vi "imprimer etiquette.vi"(0 "chaine à écrire":string="^XA\n^KL3\n^SC9600,8,N,1,,N\n^PRA\n^LL976\n^ML592\n^LH50,25\r\r^ADB,1,1^FT25,704^FDKunde:Fluid Automat. Systems GmbH^FS\r^ADB,1,1^FT50,704^FDBestellnummer:120077 / 109654     ^FS\r^ADB,1,1^FT75,704^FDKarton:1/4^FS\r^ADB,1,1^FT100,704^FDAnzahl:25/100^FS\r^ADB,1,1^FT125,704^FDIhre Art.-Nr.: MK01852 ^FS\r^ADB,1,1^FT180,704^FDVentil-Nr.:^FS\r^ADB,1,1^FT205,678^FD(P/N)^FS\r\r^FT408,40\n^BY1,2.0\n^BCI,56,N,N,N\n^FD MK01852  09 ARZAARZA 25^FS\r^AQI,1,1^FT408,10^FD MK01852  09 ARZAARZA 25^FS\r\r^A0B,18,18^FT180,568^FD ARZA6051,  ARZA6052,  ARZA6053,  ARZA6054^FS\r^A0B,18,18^FT198,568^FD ARZA6055,  ARZA6056,  ARZA6057,  ARZA6058^FS\r^A0B,18,18^FT216,568^FD ARZA6059,  ARZA6060,  ARZA6061,  ARZA6062^FS\r^A0B,18,18^FT234,568^FD ARZA6063,  ARZA6064,  ARZA6065,  ARZA6066^FS\r^A0B,18,18^FT252,568^FD ARZA6067,  ARZA6068,  ARZA6069,  ARZA6070^FS\r^A0B,18,18^FT270,568^FD ARZA6071,  ARZA6072,  ARZA6073,  ARZA6074 ^FS\r^A0B,18,18^FT288,568^FD ARZA6075 ^FS\r^A0B,18,18^FT306,568^FD ^FS\r^A0B,18,18^FT324,568^FD ^FS\r^A0B,18,18^FT242,568^FD ^FS\r\r^FT370,708\n^GB0,565,3^FS\n\n^FT501,708\n^BXB,4,0\n^FD01-223E-01-B6 F011107 18V DC 4.5W     R01159/08-01.01.01^FS\r^ADB,1,1^FT413,568^FDFAS Artikelnummer:^FS\r^AQB,1,1^FT443,568^FD01-223E-01-B6 F011107 18V DC 4.5W^FS\r^ADB,1,1^FT470,568^FDFAS Bestellnummer:^FS\r^AQB,1,1^FT500,568^FDR01159/08-01.01.01^FS\r\r^PQ1\n^XZ\r", 1 "nbr de valve":i16=10, 2 "nbr de carton":i16=1, 4 "Type de liaison":enum16{"RS232", "USB", "TCP-IP", "Aucune"}(ring)=enum."TCP-IP", 6 "Bloc Scanné":string, 7 "n°article FAS":string, 9 "sélecteur":bool, 10 "Cde_Interne":bool, 11 "error in":errorcluster caption="entrée d'erreur (pas d'erreur)", 13 "Carton Numéro":i16, 14 "fin de série ?":bool) -> (15 "error out":errorcluster caption="sortie d'erreur")   [LabVIEW 2020]
uses:
  Labview emballage/enum_ON_OFF_Lecteur.ctl
  Modules/FS/60_FS_Controles/60_FS_SetGet.ctl
  <vilib>/Instr/_visa.llb/VISA Configure Serial Port (Instr).vi
panel:
  in  "Msg Etiquette imprimée":string="L'étiquette est-elle correctement\nimprimée ?"
  out "Etiquette scanné":string
  out "Série finie":string="Il y a 1 carton(s)"
  out "Changer de carton":string="Il y a 1 carton(s)"
  out "Nbre de valve":string="pour 10 valves/blocs"
  out "Nbre de carton":string="Il y a 1 carton(s)"
  out "Carton No :":string
  out "Glissière 2":u8(slide)=100 caption="Identification terminé." scale=0.0..100.0
  in  "ré-imprimer":bool
  in  "Bouton confirmer":bool
  in  "Nom de ressource VISA USB":refnum<visa-resource-name>
  in  "Param RS232":T1={"VISA resource name"="COM4", "baud rate"=9600, "data bits"=8, "parity"=0, "stop bits"=10, "flow control"=0, "delay before read (ms)"=500} {"data bits" min=5 max=8 step=1; "parity" items=["Aucune", "Impaire", "Paire", "Marque", "Espace"]; "stop bits" items=["1.0"=10, "1.5"=15, "2.0"=20]; "flow control" items=["Aucune"=0, "XON/XOFF"=1, "RTS/CTS"=2, "DTR/DSR"=4]}
  # "LOGO FASmedic en noir et blanc"
  # "Uniquement par un responsable"
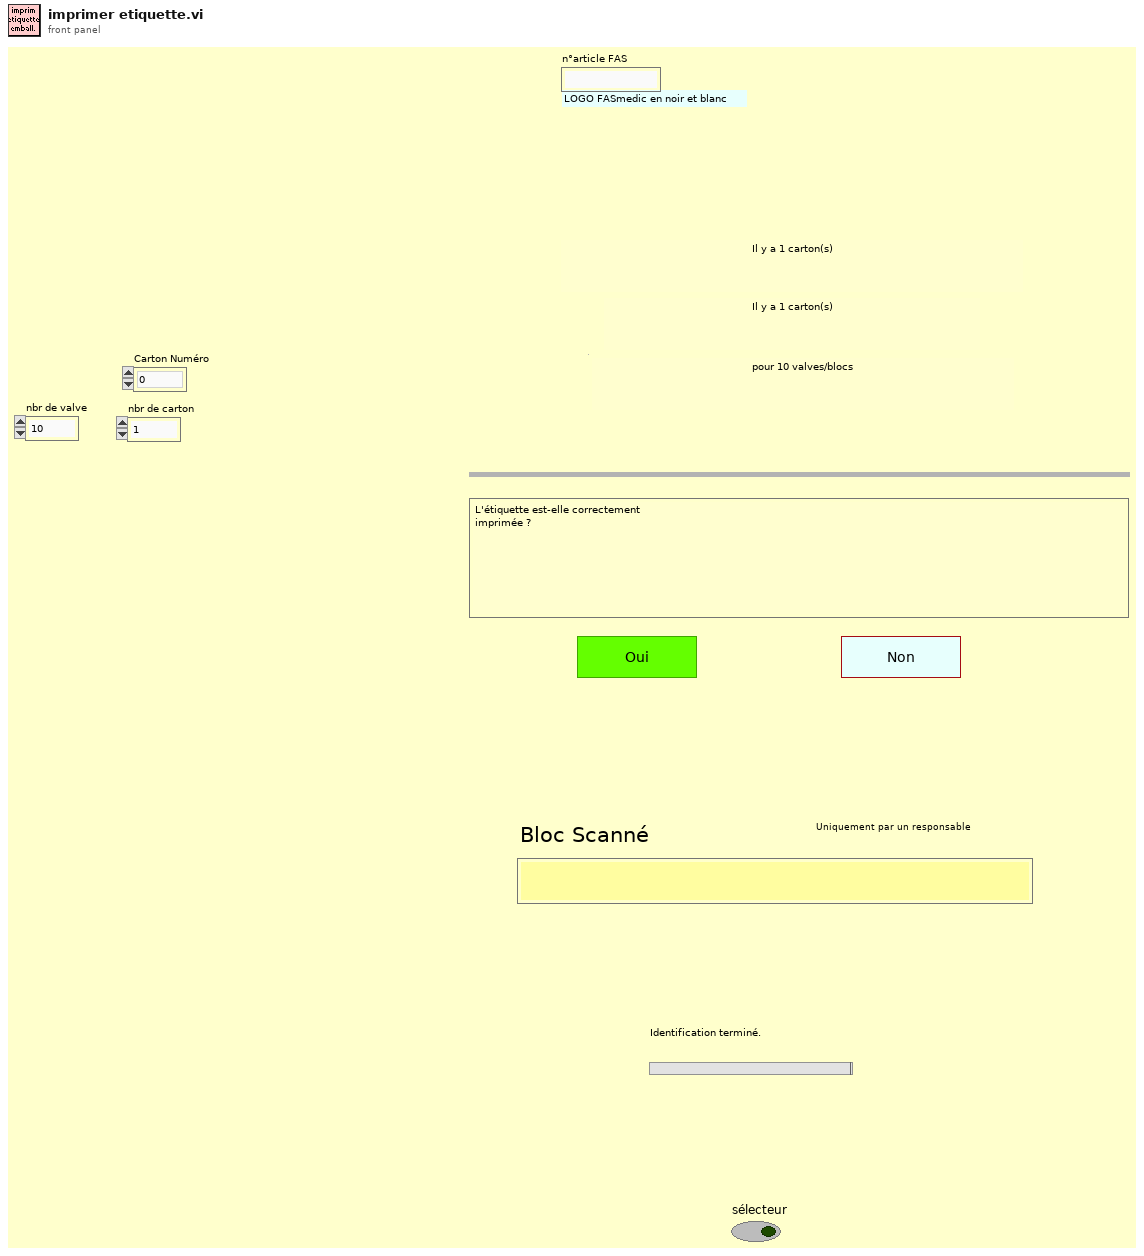
[diagram p1: front panel]
types:
  T1 = cluster{"VISA resource name":refnum<visa-resource-name>, "baud rate":u32, "data bits":u16, "parity":u16, "stop bits":u16, "flow control":u16, "delay before read (ms)":u32}
  T2 = typedef "enum_ON_OFF_Lecteur.ctl" = enum16{"ON_COURT", "OFF", "ON", "OFF (open/Close)", "ON (open/close)"}
  T3 = typedef "60_FS_SetGet.ctl" = enum16{"set", "get"}
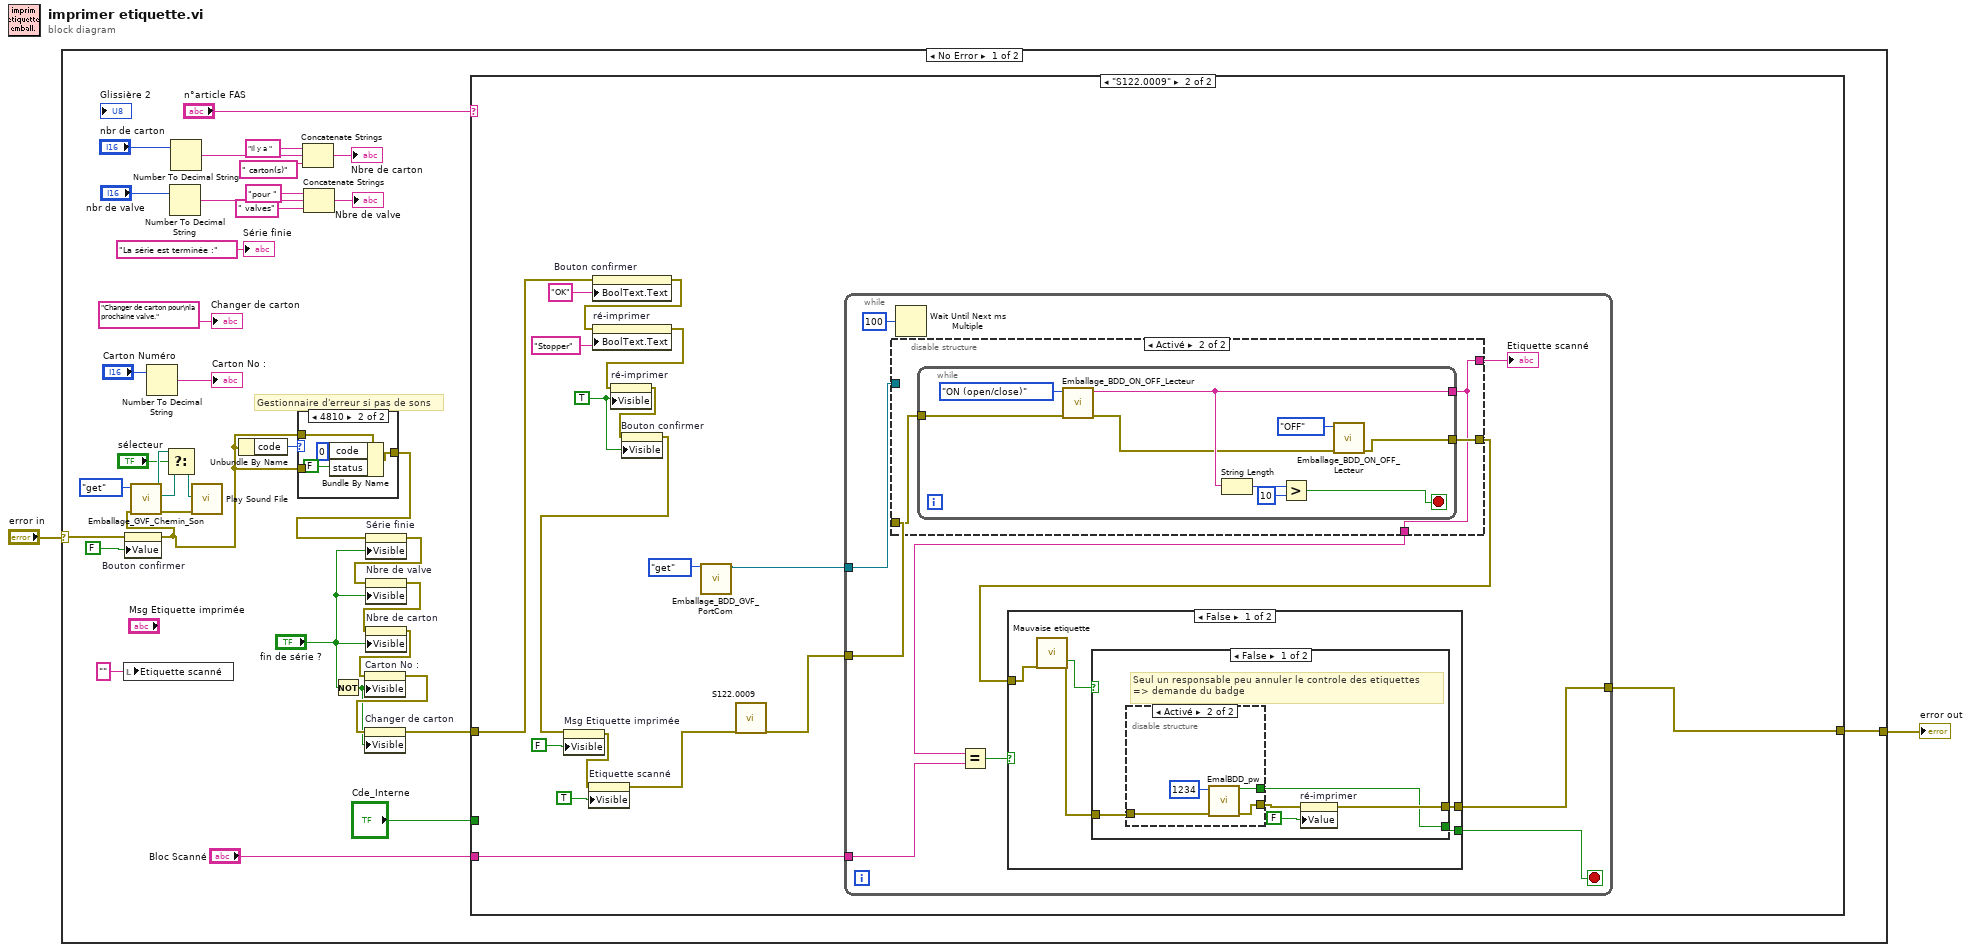
[diagram p0: block diagram]
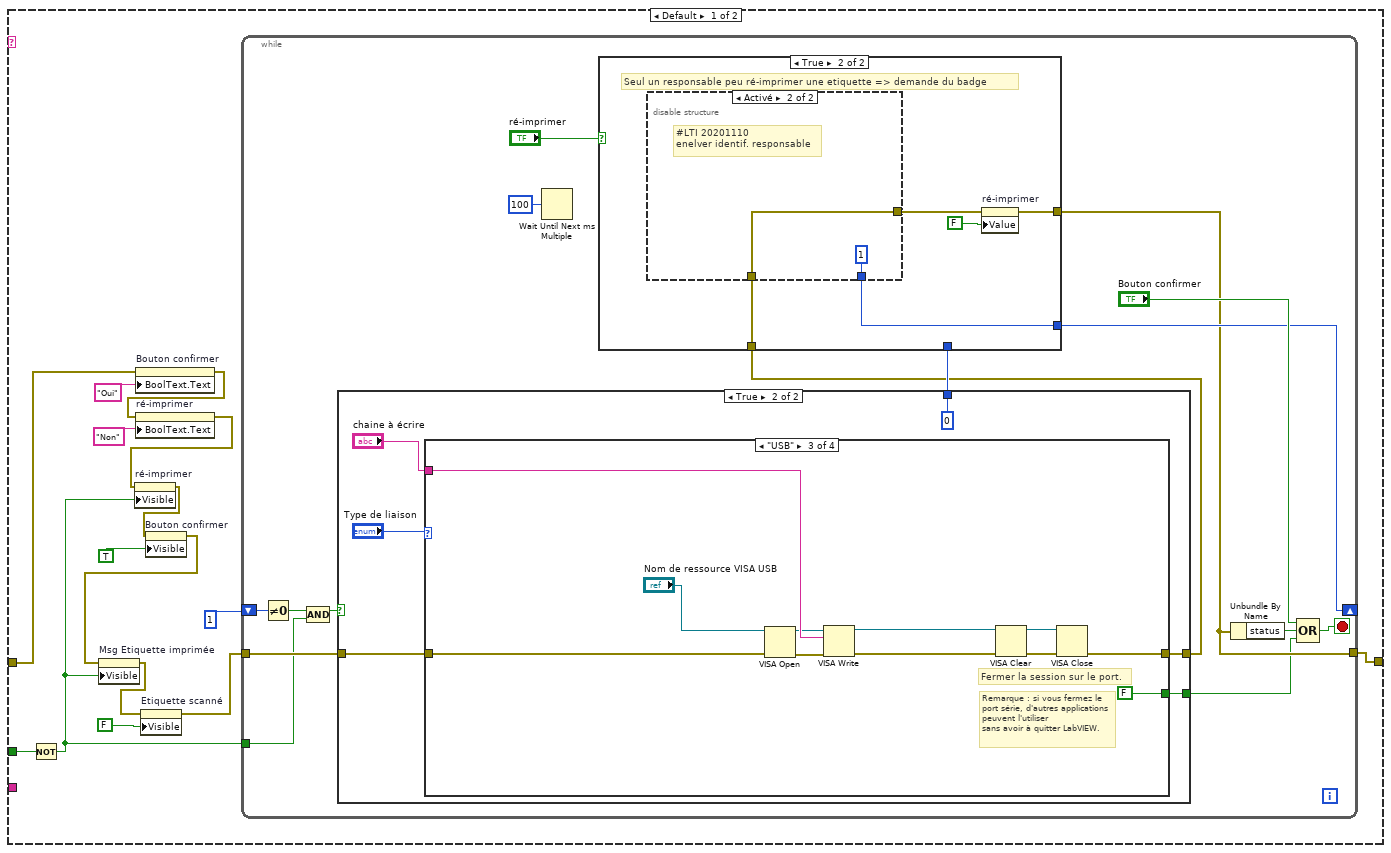
[diagram p2: hidden frame]
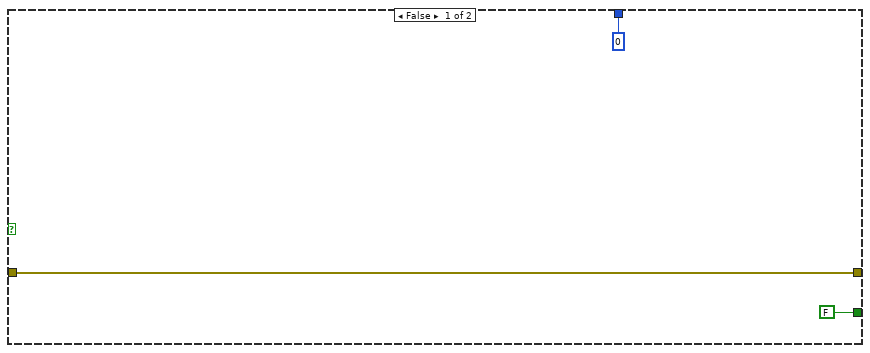
[diagram p3: hidden frame]
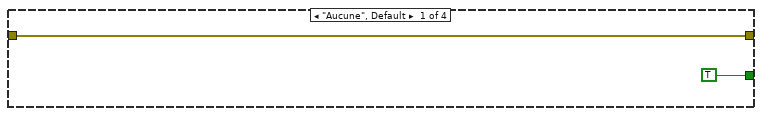
[diagram p4: hidden frame]
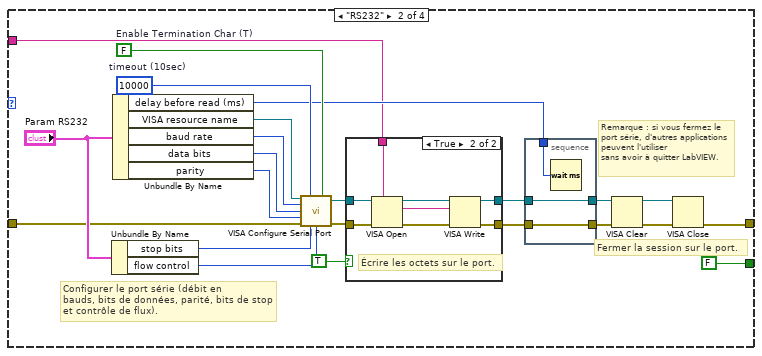
[diagram p5: hidden frame]
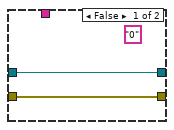
[diagram p6: hidden frame]
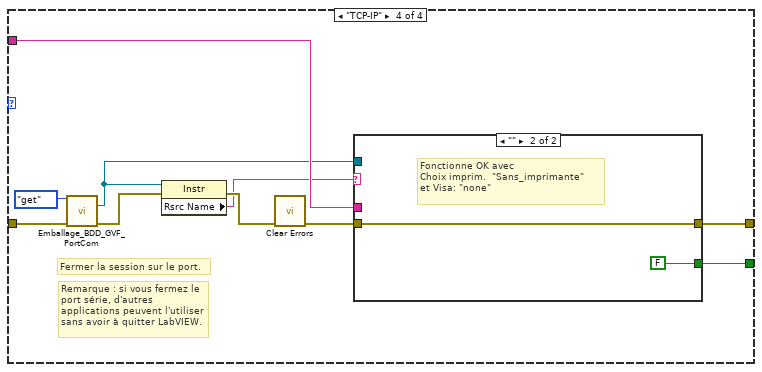
[diagram p7: hidden frame]
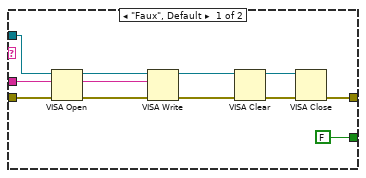
[diagram p8: hidden frame]
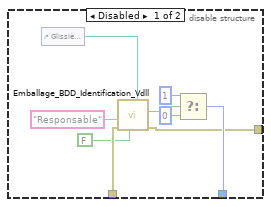
[diagram p10: hidden frame]
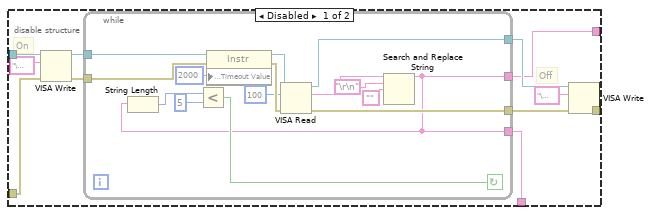
[diagram p11: hidden frame]
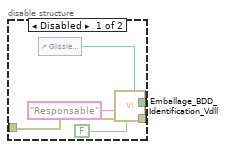
[diagram p12: hidden frame]
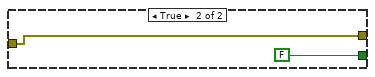
[diagram p13: hidden frame]
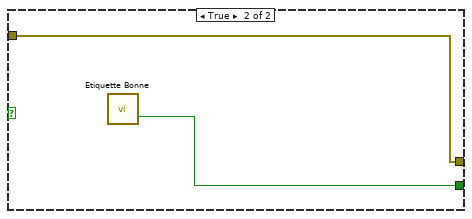
[diagram p14: hidden frame]
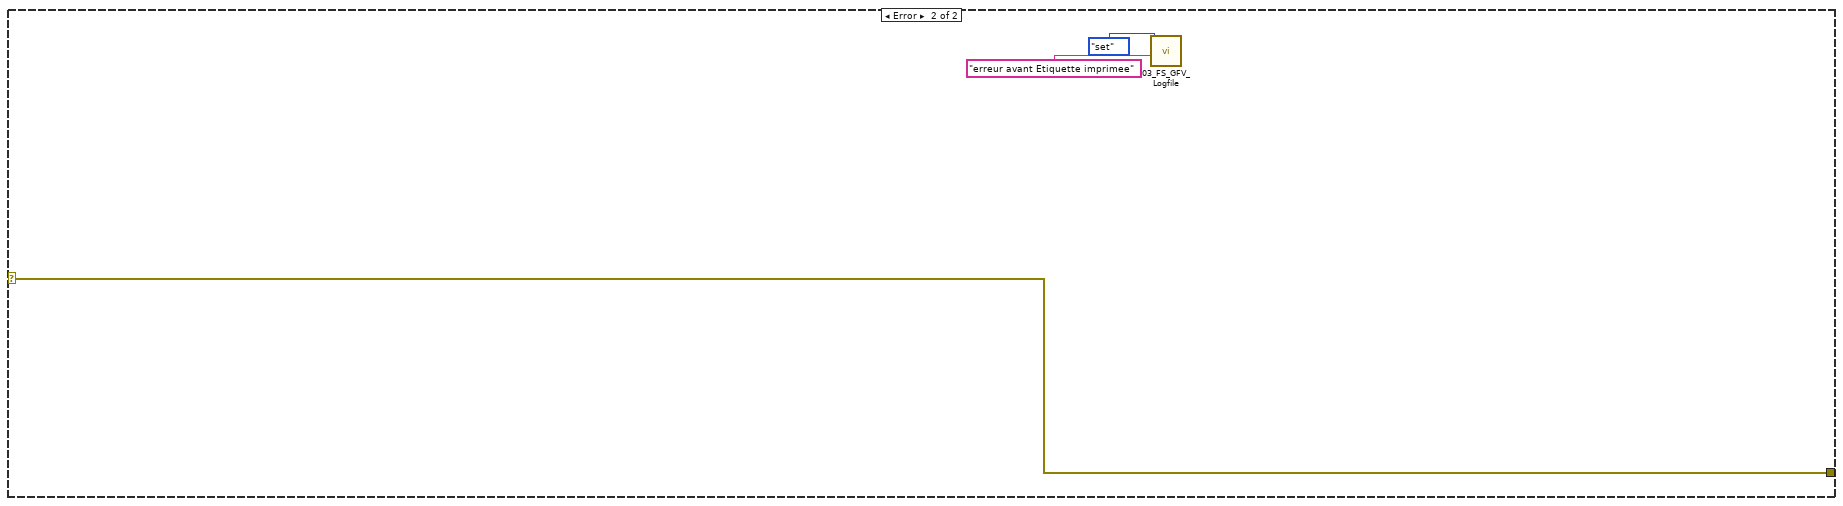
[diagram p16: hidden frame]
diagram:
  n1 = case shown="No Error" "error in" {
    selector: "error in" -> [w38 w264]
    tunnel: [w39 w264] -> w1
    frame No Error {
      # "Gestionnaire d'erreur si pas de sons"
      n2 = local write "Etiquette scanné"("" ("Numéro scanné")) -> ()
      n3 = property on="Bouton confirmer" class="Bool (strict)"(error in=w38, "Value"=FALSE ("Bouton confimer")) -> (error out=w7:errorcluster)  [unwired: 1 in, 1 out]
      n4 = call "Emballage_GVF_Chemin_Son.vi"("entrée d'erreur (pas d'erreur)"=w7, "Énum"=enum16{"get", "set"}."get") -> ("sortie d'erreur"=w8:errorcluster, "Chemin Utopia - Question.WAV"=w4:path, "Chemin The Microsoft Sound.wav"=w5:path)  [unwired: 5 in, 2 out]
      n5 = Number To Decimal String(number="Carton Numéro") -> (decimal integer string=→"Carton No :":string)  [unwired: 1 in]
      n6 = Select(t=w5, s="sélecteur", f=w4) -> (s? t:f=w6:path)
      n7 = Number To Decimal String(number="nbr de valve") -> (decimal integer string=w34:string)  [unwired: 1 in]
      n8 = Number To Decimal String(number="nbr de carton") -> (decimal integer string=w30:string)  [unwired: 1 in]
      n9 = call <vilib>:"Play Sound File.vi"("error in (no error)"=w8, "path"=w6) -> ()  [unwired: 8 in, 2 out]
      n10 = Unbundle By Name(w7) -> ("code"=w15:i32)
      n11 = case shown="4810" w15 {
        tunnel: [w257 w260] -> w14
        tunnel: w7 -> [w257 _]
        tunnel: w7 -> [_ w259]
        frame 0, Default {
        }
        frame 4810 {
          n12 = Bundle By Name(cluster=w259, "code"=0, "status"=FALSE) -> (w260:errorcluster)
        }
      }
      n13 = Concatenate Strings("Il y a ", w30, " carton(s)") -> (→"Nbre de carton":string)
      n14 = Concatenate Strings("pour ", w34, " valves") -> (→"Nbre de valve":string)
      n15 = Not(x="fin de série ?") -> (.not. x?=w19:bool)
      n16 = property on="Série finie" class="Str"(error in=w14, "Visible"="fin de série ?") -> (error out=w16:errorcluster)  [unwired: 1 in, 1 out]
      n17 = property on="Nbre de valve" class="Str"(error in=w16, "Visible"="fin de série ?") -> (error out=w26:errorcluster)  [unwired: 1 in, 1 out]
      n18 = property on="Nbre de carton" class="Str"(error in=w26, "Visible"="fin de série ?") -> (error out=w25:errorcluster)  [unwired: 1 in, 1 out]
      n19 = property on="Carton No :" class="Str"(error in=w25, "Visible"=w19) -> (error out=w23:errorcluster)  [unwired: 1 in, 1 out]
      n20 = property on="Changer de carton" class="Str"(error in=w23, "Visible"=w19) -> (error out=w22:errorcluster)  [unwired: 1 in, 1 out]
      n21 = case shown="\"S122.0009\"" "n°article FAS" {
        tunnel: [w54 w179] -> w39
        tunnel: w22 -> [w43 w172]
        tunnel: "Bloc Scanné" -> [_ w170]
        tunnel: "Cde_Interne" -> [w41 _]
        frame Default {
          n22 = Not(x=w41) -> (.not. x?=w40:bool)
          n23 = property on="Bouton confirmer" class="Bool (strict)"(error in=w43, "BoolText.Text"="Oui" ("Texte booléen.Texte")) -> (error out=w44:errorcluster)  [unwired: 1 in, 1 out]
          n24 = property on="ré-imprimer" class="Bool (strict)"(error in=w44, "BoolText.Text"="Non" ("Texte booléen.Texte")) -> (error out=w42:errorcluster)  [unwired: 1 in, 1 out]
          n25 = property on="ré-imprimer" class="Bool (strict)"(error in=w42, "Visible"=w40) -> (error out=w49:errorcluster)  [unwired: 1 in, 1 out]
          n26 = property on="Bouton confirmer" class="Bool (strict)"(error in=w49, "Visible"=TRUE) -> (error out=w47:errorcluster)  [unwired: 1 in, 1 out]
          n27 = property on="Msg Etiquette imprimée" class="Str"(error in=w47, "Visible"=w40) -> (error out=w51:errorcluster)  [unwired: 1 in, 1 out]
          n28 = property on="Etiquette scanné" class="Str"(error in=w51, "Visible"=FALSE) -> (error out=w50:errorcluster)  [unwired: 1 in, 1 out]
          n29 = while {
            tunnel: w50 -> [w69]
            tunnel: [w58] -> w54
            shift-right: [w60] -> _
            shift-left: u32 1 ("n millisecondes") -> [w62]
            tunnel: w40 -> [w55]
            stop <- w64 stop-if-true
            n30 = Not Equal To 0?(x=w62) -> (x != 0?=w63:bool)
            n31 = Compound Arithmetic op=AND(w63, w55) -> (w56:bool)
            n32 = case shown="True" w56 {
              tunnel: w69 -> [w72 w78]
              tunnel: [w72 w76] -> w59
              tunnel: [u32 0 ("n millisecondes") u32 0 ("n millisecondes")] -> w61
              tunnel: [FALSE w74] -> w57
              frame False {
              }
              frame True {
                n33 = case shown="\"USB\"" "Type de liaison" {
                  tunnel: w78 -> [w80 w88 w120 w131]
                  tunnel: [w80 w82 w121 w135] -> w76
                  tunnel: "chaine à écrire" -> [_ w87 w126 w136]
                  tunnel: [TRUE FALSE FALSE w132] -> w74
                  frame "Aucune", Default {
                  }
                  frame "RS232" {
                    w102 = FALSE  # Enable Termination Char (T)
                    w103 = u32 10000  # timeout (10sec)
                    # "Remarque : si vous fermez le port série, d'autres applications peuvent l'utiliser\nsans avoir à quitter LabVIEW."
                    # "Fermer la session sur le port."
                    # "Configurer le port série (débit en\nbauds, bits de données, parité, bits de stop\net contrôle de flux)."
                    n34 = Unbundle By Name("Param RS232") -> ("stop bits"=w96:u16, "flow control"=w95:u16)
                    n35 = Unbundle By Name("Param RS232") -> ("delay before read (ms)"=w91:u32, "VISA resource name"=w101:refnum<visa-resource-name>, "baud rate"=w100:u32, "data bits"=w99:u16, "parity"=w98:u16)
                    n36 = call-poly "VISA Configure Serial Port"("VISA resource name"=w101, "timeout (10sec)"=w103, "Enable Termination\nChar (T)"=w102, "baud rate (9600)"=w100, "data bits (8)"=w99, "parity (0:none)"=w98, "error in (no error)"=w88, "stop bits (10: 1 bit)"=w96, "flow control (0:none)"=w95) -> ("VISA resource name out"=w90:refnum<visa-resource-name>, "error out"=w89:errorcluster)  [unwired: 5 in]
                    n37 = case shown="True" TRUE {
                      tunnel: [w108 w115] -> w94
                      tunnel: w90 -> [w107 w114]
                      tunnel: w89 -> [w108 w110]
                      tunnel: [w107 w113] -> w93
                      tunnel: w87 -> [_ w112]
                      frame False {
                        (unwired) "0" ("string to write")
                      }
                      frame True {
                        # "Écrire les octets sur le port."
                        n38 = VISA Open(error in (no error)=w110, VISA resource name=w114) -> (VISA resource name=w111:refnum<visa-resource-name>, error out=w109:errorcluster)  [unwired: 3 in]
                        n39 = VISA Write(VISA resource name=w111, write buffer=w112, error in (no error)=w109) -> (VISA resource name out=w113:refnum<visa-resource-name>, error out=w115:errorcluster)  [unwired: 1 out]
                      }
                    }
                    n40 = stacked-sequence {
                      tunnel: w94 -> [w106]
                      tunnel: [w106] -> w84
                      tunnel: w93 -> [w105]
                      tunnel: [w105] -> w83
                      tunnel: w91 -> [w104]
                      frame #0 {
                        n41 = Wait (ms)(milliseconds to wait=w104) -> ()  [unwired: 1 out]
                      }
                    }
                    n42 = VISA Clear(VISA resource name=w83, error in (no error)=w84) -> (VISA resource name out=w85:refnum<visa-resource-name>, error out=w86:errorcluster)
                    n43 = VISA Close(VISA resource name=w85, error in (no error)=w86) -> (error out=w82:errorcluster)
                  }
                  frame "USB" {
                    # "Remarque : si vous fermez le port série, d'autres applications peuvent l'utiliser\nsans avoir à quitter LabVIEW."
                    # "Fermer la session sur le port."
                    n44 = VISA Open(error in (no error)=w120, VISA resource name="Nom de ressource VISA USB") -> (VISA resource name=w118:refnum<visa-resource-name>, error out=w117:errorcluster)  [unwired: 3 in]
                    n45 = VISA Write(VISA resource name=w118, write buffer=w126, error in (no error)=w117) -> (VISA resource name out=w122:refnum<visa-resource-name>, error out=w123:errorcluster)  [unwired: 1 out]
                    n46 = VISA Clear(VISA resource name=w122, error in (no error)=w123) -> (VISA resource name out=w124:refnum<visa-resource-name>, error out=w125:errorcluster)
                    n47 = VISA Close(VISA resource name=w124, error in (no error)=w125) -> (error out=w121:errorcluster)
                  }
                  frame "TCP-IP" {
                    # "Remarque : si vous fermez le port série, d'autres applications peuvent l'utiliser\nsans avoir à quitter LabVIEW."
                    # "Fermer la session sur le port."
                    n48 = call "Emballage_BDD_GVF_PortCom.vi"("Énum"=enum16{"get", "set"}."get", "Error in"=w131) -> ("PortCom imprimante OUT"=w128:refnum<visa-resource-name>, "Error out"=w130:errorcluster)  [unwired: 7 in, 5 out]
                    n49 = property class="Instr"(reference=w128, error in=w130) -> (error out=w134:errorcluster, "Rsrc Name"=w127:string)  [unwired: 1 out]
                    n50 = call <vilib>:"Clear Errors.vi"("error in (no error)"=w134) -> ("error out"=w133:errorcluster)  [unwired: 5 in, 1 out]
                    n51 = case shown="\"\"" w127 {
                      tunnel: w136 -> [w147 _]
                      tunnel: [w142 w149] -> w135
                      tunnel: w133 -> [w140 w149]
                      tunnel: w128 -> [w138 _]
                      tunnel: [FALSE FALSE] -> w132
                      frame "Faux", Default {
                        n52 = VISA Open(error in (no error)=w140, VISA resource name=w138) -> (VISA resource name=w141:refnum<visa-resource-name>, error out=w139:errorcluster)  [unwired: 3 in]
                        n53 = VISA Write(VISA resource name=w141, write buffer=w147, error in (no error)=w139) -> (VISA resource name out=w143:refnum<visa-resource-name>, error out=w144:errorcluster)  [unwired: 1 out]
                        n54 = VISA Clear(VISA resource name=w143, error in (no error)=w144) -> (VISA resource name out=w145:refnum<visa-resource-name>, error out=w146:errorcluster)
                        n55 = VISA Close(VISA resource name=w145, error in (no error)=w146) -> (error out=w142:errorcluster)
                      }
                      frame "" {
                        # "Fonctionne OK avec \nChoix imprim.  \"Sans_imprimante\"\net Visa: \"none\""
                      }
                    }
                  }
                }
              }
            }
            n56 = Wait Until Next ms Multiple(millisecond multiple=u32 100 ("n millisecondes")) -> ()  [unwired: 1 out]
            n57 = case shown="True" "ré-imprimer" {
              tunnel: w61 -> [w151 _]
              tunnel: [w151 w156] -> w60
              tunnel: w59 -> [w150 w155]
              tunnel: [w150 w154] -> w58
              frame False {
              }
              frame True {
                # "Seul un responsable peu ré-imprimer une etiquette => demande du badge"
                n58 = disable-structure shown="Activé" {
                  disable-tunnel: [w162 u32 1 ("cas faux")] -> w156
                  disable-tunnel: w155 -> [w160 w166]
                  disable-tunnel: [w157 w166] -> w153
                  frame Disabled {
                    n59 = control-ref of="Glissière 2"() -> (w158:refnum<vi>)
                    n60 = call "Emballage_BDD_Identification_Vdll.vi"("Glissière"=w158, "lecture seul possible ?"=FALSE, "error in"=w160, "Posage choisi"="Responsable" ("Posage choissi")) -> ("error Out"=w157:errorcluster, "OK"=w164:bool)  [unwired: 3 in, 3 out]
                    n61 = Select(t=u32 1 ("n millisecondes"), s=w164, f=u32 0 ("cas faux")) -> (s? t:f=w162:u32)
                  }
                  frame Enabled {
                    # "#LTI 20201110\nenelver identif. responsable"
                  }
                }
                n62 = property on="ré-imprimer" class="Bool (strict)"(error in=w153, "Value"=FALSE ("ré-imprimer")) -> (error out=w154:errorcluster)  [unwired: 1 in, 1 out]
              }
            }
            n63 = Unbundle By Name(w58) -> ("status"=w66:bool)
            n64 = Compound Arithmetic op=OR("Bouton confirmer", w66, w57) -> (w64:bool)
          }
        }
        frame "S122.0009" {
          w178 = TRUE ("Visible")
          n65 = property on="Bouton confirmer" class="Bool (strict)"(error in=w172, "BoolText.Text"="OK" ("Texte booléen.Texte")) -> (error out=w173:errorcluster)  [unwired: 1 in, 1 out]
          n66 = property on="ré-imprimer" class="Bool (strict)"(error in=w173, "BoolText.Text"="Stopper" ("Texte booléen.Texte")) -> (error out=w171:errorcluster)  [unwired: 1 in, 1 out]
          n67 = property on="ré-imprimer" class="Bool (strict)"(error in=w171, "Visible"=w178) -> (error out=w177:errorcluster)  [unwired: 1 in, 1 out]
          n68 = property on="Bouton confirmer" class="Bool (strict)"(error in=w177, "Visible"=w178) -> (error out=w176:errorcluster)  [unwired: 1 in, 1 out]
          n69 = property on="Msg Etiquette imprimée" class="Str"(error in=w176, "Visible"=FALSE) -> (error out=w182:errorcluster)  [unwired: 1 in, 1 out]
          n70 = property on="Etiquette scanné" class="Str"(error in=w182, "Visible"=TRUE) -> (error out=w181:errorcluster)  [unwired: 1 in, 1 out]
          n71 = call "Emballage_BDD_GVF_PortCom.vi"("Énum"=enum16{"get", "set"}."get") -> ("PortCom Scanner"=w168:refnum<visa-resource-name>)  [unwired: 8 in, 6 out]
          n72 = call "S122.0009"("error in (no error)"=w181) -> ("error out"=w180:errorcluster)  [unwired: 17 in, 1 out]
          n73 = while {
            tunnel: w168 -> [w194]
            tunnel: w180 -> [w193]
            tunnel: [w187] -> w179
            tunnel: w170 -> [w192]
            stop <- w188 stop-if-true
            n74 = disable-structure shown="Activé" {
              disable-tunnel: w194 -> [w205 _]
              disable-tunnel: w193 -> [w204 w223]
              disable-tunnel: [w197 w221] -> w191
              disable-tunnel: [w196 w222] -> w186
              disable-tunnel: [w195 w221] -> w185
              frame Disabled {
                # "Off"
                # "On"
                n75 = VISA Write(VISA resource name=w205, write buffer="\u0002", error in (no error)=w204) -> (VISA resource name out=w202:refnum<visa-resource-name>, error out=w203:errorcluster)  [unwired: 1 out]
                n76 = while {
                  tunnel: [w220] -> w198
                  tunnel: w203 -> [w212]
                  tunnel: w202 -> [w211]
                  tunnel: [w207] -> w199
                  tunnel: [w206] -> w197
                  tunnel: [w206] -> w195
                  stop <- w208 continue-if-true
                  n77 = property class="Instr"(reference=w211, error in=w212, "General Settings:Timeout Value"=u32 2000 ("Tmo Value")) -> (reference out=w218:refnum<visa-resource-name>, error out=w219:errorcluster)
                  n78 = VISA Read(VISA resource name=w218, byte count=u32 100 ("byte count (0)"), error in (no error)=w219) -> (VISA resource name out=w207:refnum<visa-resource-name>, read buffer=w215:string, error out=w220:errorcluster)  [unwired: 1 out]
                  n79 = Search and Replace String(input string=w215, search string="\r\n", replace string="") -> (result string=w206:string)  [unwired: 5 in, 3 out]
                  n80 = String Length(string=w206) -> (length=w210:i32)
                  n81 = Less?(x=w210, y=5) -> (x < y?=w208:bool)
                }
                n82 = VISA Write(VISA resource name=w199, write buffer="\u0003", error in (no error)=w198) -> (error out=w196:errorcluster)  [unwired: 2 out]
              }
              frame Enabled {
                n83 = while {
                  tunnel: w223 -> [w231]
                  tunnel: [w228] -> w221
                  tunnel: [w226] -> w222
                  stop <- w227 stop-if-true
                  n84 = call "Emballage_BDD_ON_OFF_Lecteur.vi"("Error in"=w231, "ON/OFF lecteur"=enum_ON_OFF_Lecteur."ON (open/close)") -> ("Error out"=w225:errorcluster, "Etiquette scanné"=w228:string)  [unwired: 7 in, 1 out]
                  n85 = String Length(string=w228) -> (length=w229:i32)
                  n86 = Greater?(x=w229, y=10) -> (0:w227:bool)
                  n87 = call "Emballage_BDD_ON_OFF_Lecteur.vi"("Error in"=w225, "ON/OFF lecteur"=enum_ON_OFF_Lecteur."OFF") -> ("Error out"=w226:errorcluster)  [unwired: 7 in, 2 out]
                }
              }
            }
            "Etiquette scanné" <- w185
            n88 = Wait Until Next ms Multiple(millisecond multiple=u32 100 ("n millisecondes")) -> ()  [unwired: 1 out]
            n89 = Equal?(x=w191, y=w192) -> (x = y?=w189:bool)
            n90 = case shown="False" w189 {
              tunnel: [w233 w256] -> w188
              tunnel: [w235 w255] -> w187
              tunnel: w186 -> [w234 w255]
              frame False {
                n91 = call "Mauvaise etiquette"("error in (no error)"=w234) -> ("OK"=w237:bool, "error out"=w236:errorcluster)  [unwired: 17 in]
                n92 = case shown="False" w237 {
                  tunnel: w236 -> [w242 w254]
                  tunnel: [w241 w254] -> w235
                  tunnel: [w238 FALSE ("OK")] -> w233
                  frame False {
                    # "Seul un responsable peu annuler le controle des etiquettes \n=> demande du badge"
                    n93 = disable-structure shown="Activé" {
                      disable-tunnel: w242 -> [w247 w251]
                      disable-tunnel: [w244 w250] -> w240
                      disable-tunnel: [w243 w249] -> w238
                      frame Disabled {
                        n94 = control-ref of="Glissière 2"() -> (w245:refnum<vi>)
                        n95 = call "Emballage_BDD_Identification_Vdll.vi"("Glissière"=w245, "lecture seul possible ?"=FALSE, "error in"=w247, "Posage choisi"="Responsable" ("Posage choissi")) -> ("error Out"=w244:errorcluster, "OK"=w243:bool)  [unwired: 3 in, 3 out]
                      }
                      frame Enabled {
                        n96 = call "EmalBDD_pw.vi"("Error in"=w251, "PWattendu"=u32 1234) -> ("Error Out"=w250:errorcluster, "pwOK?"=w249:bool)  [unwired: 8 in]
                      }
                    }
                    n97 = property on="ré-imprimer" class="Bool (strict)"(error in=w240, "Value"=FALSE ("ré-imprimer")) -> (error out=w241:errorcluster)  [unwired: 1 in, 1 out]
                  }
                  frame True {
                  }
                }
              }
              frame True {
                n98 = call "Etiquette Bonne"() -> ("OK"=w256:bool)  [unwired: 18 in, 1 out]
              }
            }
          }
        }
      }
      "Changer de carton" <- "Changer de carton pour\nla prochaine valve." ("Changer de carton")
      "Série finie" <- "La série est terminée :" ("Changer de carton 2")
    }
    frame Error {
      n99 = call "03_FS_GFV_Logfile.vi"("Chaîne"="erreur avant Etiquette imprimee", "States"=60_FS_SetGet."set") -> ()  [unwired: 8 in, 2 out]
    }
  }
  "error out" <- w1
